vi "DefenseWall.vi"(0 "object in":refnum<class "DefendAreaTactic.lvclass">, 2 "Robot":refnum<class "Robot.lvclass">, 3 "Game in":refnum<class "Game.lvclass">, 5 "error in (no error)":errorcluster, 9 "number of defenders":i32) -> (14 "object out":refnum<class "DefendAreaTactic.lvclass">, 16 "Robot 2":refnum<class "Robot.lvclass">, 19 "error out":errorcluster)   [LabVIEW 2024, in "DefendAreaTactic.lvclass"]
uses:
  DefendAreaTactic.lvclass
  Game_class/Game.lvclass
  Robot_class/Robot.lvclass
  Game_class/Game.lvclass/Game.ctl
  Team_class/Team.lvclass/Team.ctl
  Robot_class/Robot.lvclass/Robot.ctl
  Robot_class/Write dest_x.vi
  Robot_class/Write dest_y.vi
  Robot_class/Write dest_orientation.vi
  Game_class/Read KeeperTeam.vi
  Game_class/Read DefensiveTeam.vi
  Team_class/Read RobotRef.vi
  Robot_class/Read dest_x.vi
  Ally_class/Ally.lvclass
  C:/Users/ROBOIME2/Documents/SSL ROBOIME/SSL_AI/Team_class/Team.lvclass
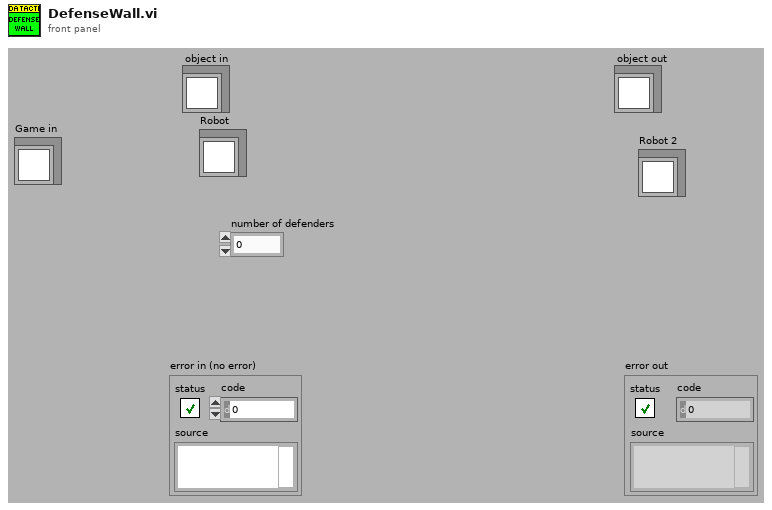
[diagram p1: front panel]
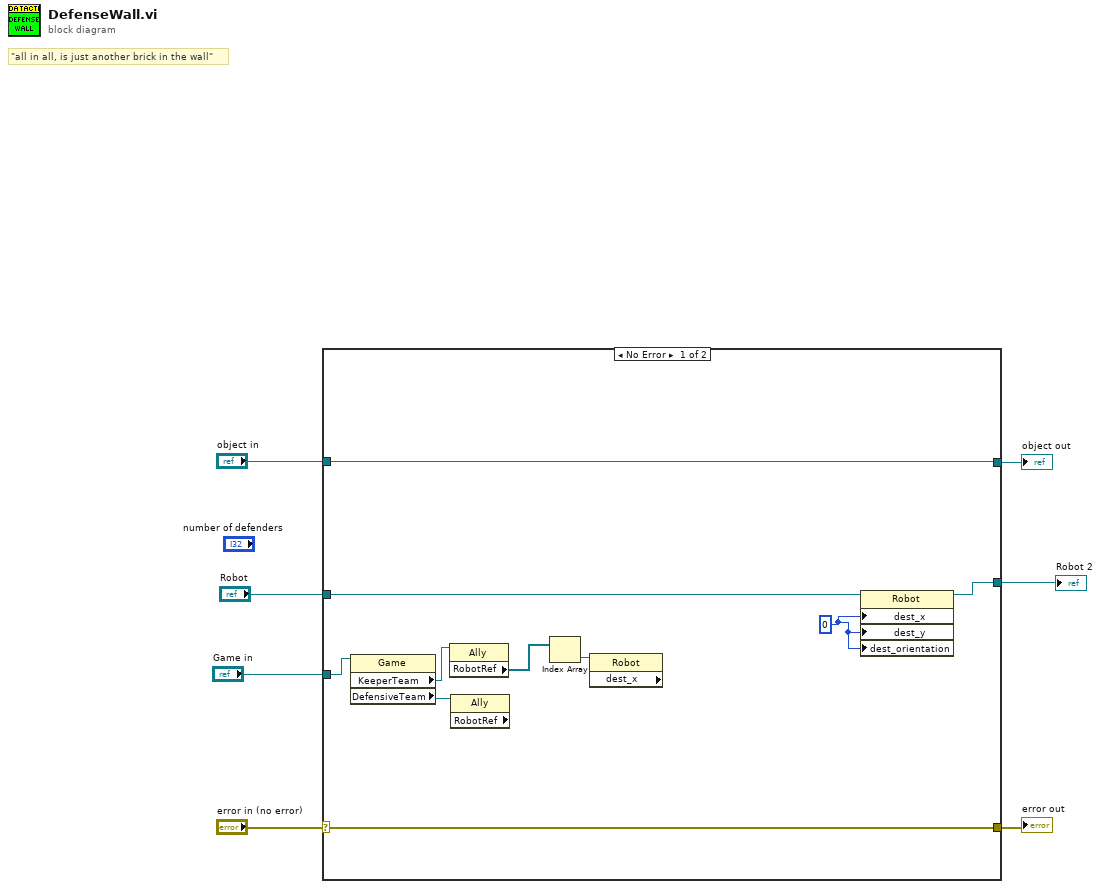
[diagram p0: block diagram]
diagram:
  # "\"all in all, is just another brick in the wall\""
  n1 = case shown="No Error" "error in (no error)" {
    selector: "error in (no error)" -> [w17 w20]
    tunnel: [w17 w20] -> w6
    tunnel: [w14 w19] -> w4
    tunnel: "object in" -> [w14 w19]
    tunnel: "Game in" -> [w16 _]
    tunnel: [w13 w18] -> w2
    tunnel: "Robot" -> [w12 w18]
    frame No Error {
      w8 = 0
      n2 = property class="Game"(reference=w16) -> ("KeeperTeam"=w11:refnum<class "Ally.lvclass">, "DefensiveTeam"=w15:refnum<class "Ally.lvclass">)  [unwired: 1 in, 2 out]
      n3 = property class="Ally"(reference=w11) -> ("RobotRef"=w10:refnum<class "Robot.lvclass">[])  [unwired: 1 in, 2 out]
      n4 = property class="Ally" props=["RobotRef"](reference=w15) -> ()  [unwired: 1 in, 3 out]
      n5 = Index Array(array=w10) -> (element=w9:refnum<class "Robot.lvclass">)  [unwired: 1 in]
      n6 = property class="Robot" props=["dest_x"](reference=w9) -> ()  [unwired: 1 in, 3 out]
      n7 = property class="Robot"(reference=w12, "dest_x"=w8, "dest_y"=w8, "dest_orientation"=w8) -> (reference out=w13:refnum<class "Robot.lvclass">)  [unwired: 1 in, 1 out]
    }
    frame Error {
    }
  }
  "error out" <- w6
  "object out" <- w4
  "Robot 2" <- w2
